vi "Query FDT Memory.vi"(0 "VISA resource name":refnum<visa-resource-name>, 11 "error in (no error)":errorcluster) -> (4 "VISA resource name out":refnum<visa-resource-name>, 6 "Memory Used":i32, 8 "Memory Available":i32, 10 "Table Array":string[](array[string]), 15 "error out":errorcluster)   [LabVIEW 2014, in "Agilent U2000 Series.lvlib"]
doc: "Queries the status of frequency dependent tables in instrument memory."
uses:
  Agilent U2000 Series.lvlib
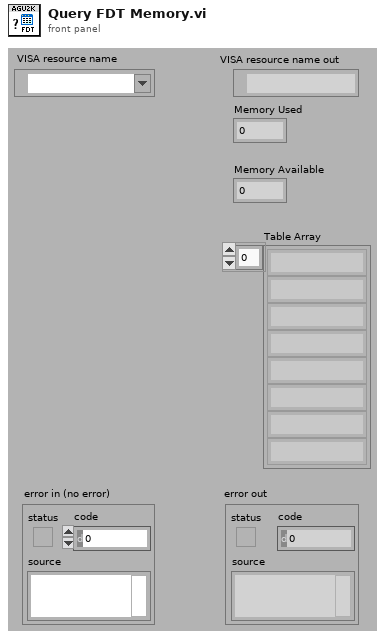
[diagram p1: front panel]
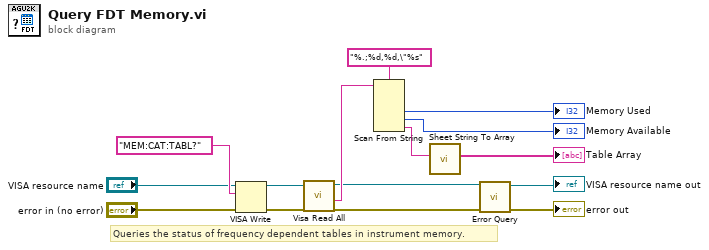
[diagram p0: block diagram]
diagram:
  # "Queries the status of frequency dependent tables in instrument memory."
  n1 = VISA Write(VISA resource name="VISA resource name", write buffer="MEM:CAT:TABL?", error in (no error)="error in (no error)") -> (VISA resource name out=w9:refnum<visa-resource-name>, error out=w8:errorcluster)  [unwired: 1 out]
  n2 = call "Visa Read All.vi"("error in (no error)"=w8, "VISA resource name"=w9) -> ("error out"=w1:errorcluster, "Read Buffer"=w7:string, "VISA resource name out"=w4:refnum<visa-resource-name>)  [unwired: 7 out]
  n3 = Scan From String(format string="%.;%d,%d,\"%s", input string=w7) -> (output 1=→"Memory Used":i32, output 2=→"Memory Available":i32, output 3=w6:string)  [unwired: 2 in, 6 out]
  n4 = call "Sheet String To Array.vi"("Sheet String"=w6) -> ("Table Array"=→"Table Array":string[])  [unwired: 10 out]
  n5 = call "Error Query.vi"("error in (no error)"=w1, "VISA resource name"=w4) -> ("error out"=→"error out":errorcluster, "VISA resource name out"=→"VISA resource name out":refnum<visa-resource-name>)  [unwired: 8 out]
